vi "runtime io test.vi"() -> ()   [LabVIEW 2013, in "processing plugin tests.lvlib"]
uses:
  processing plugin tests.lvlib
  module/execution/tag bus processing plugin module.lvclass
  <vilib>/NI/Tag Bus/tag/tag descriptor.lvclass/tag descriptor.ctl
  <vilib>/NI/Tag Bus/table/data polymorphs/write one/write Double.vi
  <vilib>/NI/Tag Bus/table/data polymorphs/read one/read Double.vi
  <vilib>/NI/Tag Bus/tag/read tag name.vi
  <vilib>/NI/Tag Bus/tag/read data type.vi
  <vilib>/NI/Tag Bus/dictionary/data dictionary.lvclass
  <vilib>/NI/Tag Bus Module Framework/channel/TBM channel.lvclass
  <vilib>/NI/Tag Bus/table/data table.lvlib
panel:
  out "inputs changed?":bool
  out "no error":errorcluster
  # "This is expected to remain false until you write code for input"
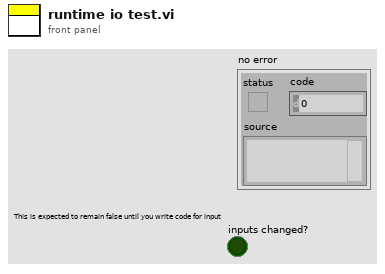
[diagram p1: front panel]
types:
  T1 = typedef "tag bus processing plugin module configuration.lvclass/processing channels.ctl" = cluster{"parameter":refnum<class "TBM channel.lvclass">, "result":refnum<class "TBM channel.lvclass">}
  T2 = typedef "tag bus.lvlib/tag descriptor.lvclass/Data Type.ctl" = enum16{"Double", "Single", "I64", "I32", "I16", "I8", "U64", "U32", "U16", "U8", "Boolean", "String", "Array of Double", "Array of Single", "Array of I64", "Array of I32", "Array of I16", "Array of I8", "Array of U64", "Array of U32", "Array of U16", "Array of U8", "Array of Boolean", "Array of String"}
  T3 = typedef "TBM channel.lvclass/data tables.ctl" = cluster{"input data":T4, "processing parameter":T4, "processing result":T4, "output data":T4}
  T4 = typedef "tag bus.lvlib/dictionary table pair.ctl" = cluster{"data dictionary":refnum<class "data dictionary.lvclass">, "data table":T5}
  T5 = typedef "tag bus.lvlib/data table.lvlib/data table.ctl" = cluster{"Double":dbl[], "Single":sgl[], "I64":i64[], "I32":i32[], "I16":i16[], "I8":i8[], "U64":u64[], "U32":u32[], "U16":u16[], "U8":u8[], "Boolean":bool[], "String":string[], "Array of Double":cluster{"DBL Array":dbl[]}[], "Array of Single":cluster{"SGL Array":sgl[]}[], "Array of I64":cluster{"I64 Array":i64[]}[], "Array of I32":cluster{"I32 Array":i32[]}[], "Array of I16":cluster{"I16 Array":i16[]}[], "Array of I8":cluster{"I8 Array":i8[]}[], "Array of U64":cluster{"U64 Array":u64[]}[], "Array of U32":cluster{"U32 Array":u32[]}[], "Array of U16":cluster{"U16 Array":u16[]}[], "Array of U8":cluster{"U8 Array":u8[]}[], "Array of Boolean":cluster{"Boolean Array":bool[]}[], "Array of String":cluster{"String Array":string[]}[]}
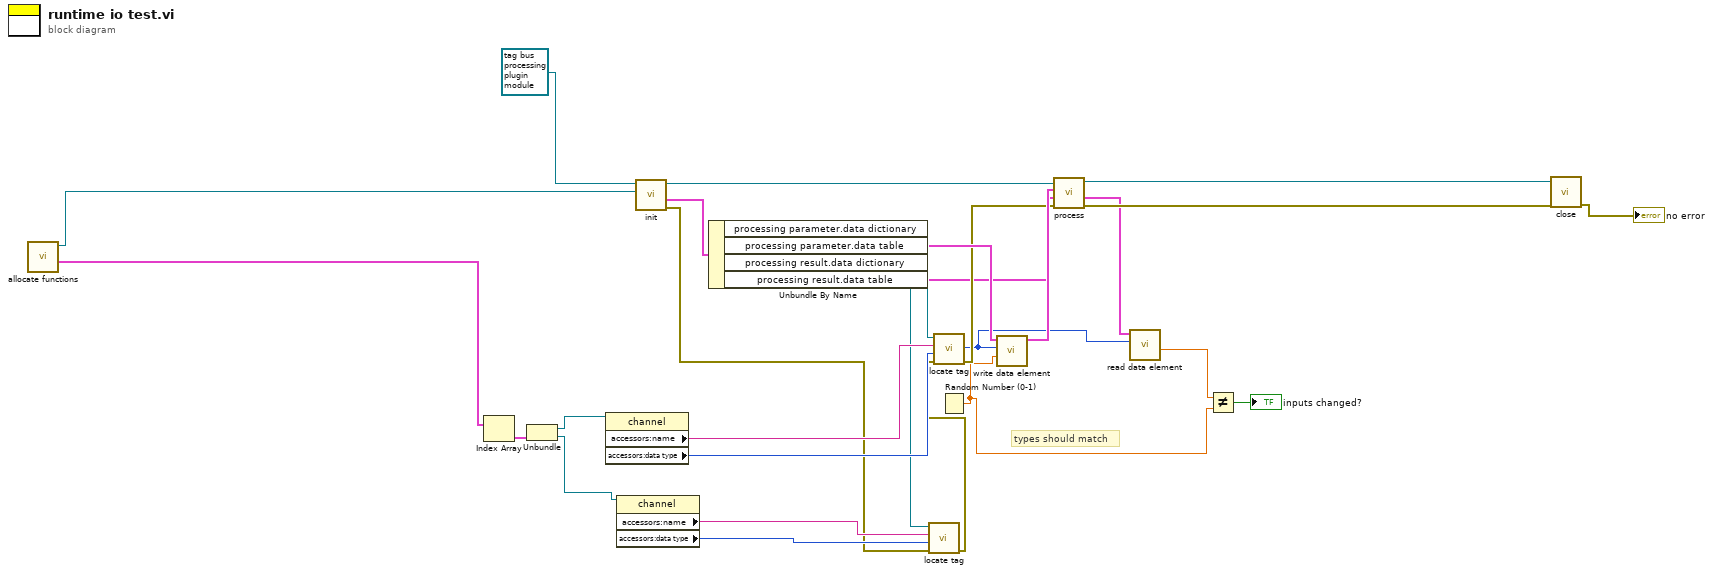
[diagram p0: block diagram]
diagram:
  # "types should match"
  n1 = call "allocate functions.vi"() -> ("functions"=w5:T1[], "tag bus processing plugin module configuration out"=w1:refnum<class "tag bus processing plugin module configuration.lvclass">)  [unwired: 9 in, 1 out]
  n2 = Index Array(array=w5) -> (element=w4:T1)  [unwired: 1 in]
  n3 = Unbundle(w4) -> ("parameter"=w3:refnum<class "TBM channel.lvclass">, "result"=w2:refnum<class "TBM channel.lvclass">)
  n4 = property class="channel"(reference=w3) -> ("accessors:name"=w21:string, "accessors:data type"=w22:T2)  [unwired: 1 in, 2 out]
  n5 = property class="channel"(reference=w2) -> ("accessors:name"=w12:string, "accessors:data type"=w11:T2)  [unwired: 1 in, 2 out]
  n6 = call-dynamic "init.vi"("TBM module configuration in"=w1, "tag bus configurable plugin module in"=refnum<class "tag bus processing plugin module.lvclass"> refnum ("tag bus configurable plugin module")) -> ("error out"=w10:errorcluster, "data allocations"=w24:T3, "tag bus configurable plugin module out"=w25:refnum<class "tag bus processing plugin module.lvclass">)  [unwired: 6 in, 1 out]
  n7 = Unbundle By Name(w24) -> ("processing parameter.data dictionary"=w23:refnum<class "data dictionary.lvclass">, "processing parameter.data table"=w20:T5, "processing result.data dictionary"=w13:refnum<class "data dictionary.lvclass">, "processing result.data table"=w6:T5)
  n8 = call <vilib>:"locate tag.vi"("error in"=w10, "data type"=w11, "name"=w12, "data dictionary in"=w13) -> ("error out"=w9:errorcluster)  [unwired: 5 in, 2 out]
  n9 = call <vilib>:"locate tag.vi"("error in"=w9, "data type"=w22, "name"=w21, "data dictionary in"=w23) -> ("error out"=w18:errorcluster, "index"=w17:i32)  [unwired: 5 in, 1 out]
  n10 = Random Number (0-1)() -> (number: 0 to 1=w16:dbl)
  n11 = call-poly <vilib>:"write data element.vi"("value"=w16, "index"=w17, "data table in"=w20) -> ("data table out"=w19:T5)  [unwired: 8 in]
  n12 = call-dynamic "process.vi"("error in"=w18, "result allocation"=w6, "data to process"=w19, "module in"=w25) -> ("error out"=w26:errorcluster, "result data"=w7:T5, "module out"=w27:refnum<class "tag bus processing plugin module.lvclass">)  [unwired: 4 in, 1 out]
  n13 = call-poly <vilib>:"read data element.vi"("index"=w17, "data table in"=w7) -> ("value"=w15:dbl)  [unwired: 8 in, 1 out]
  n14 = Not Equal?(x=w15, y=w16) -> (x != y?=→"inputs changed?":bool)
  n15 = call-dynamic "close.vi"("error in"=w26, "tag bus configurable plugin module in"=w27) -> ("error out"=→"no error":errorcluster)  [unwired: 9 in]
